vi "open-res-ra.vi"(7 "res-ra config":T1={"resource-type"="battery", "ra-ip"="127.0.0.1", "write-port"=32011, "listen-port"=32001}) -> (0 "error out":errorcluster, 5 "connection ID":refnum<k16>)   [LabVIEW 2021]
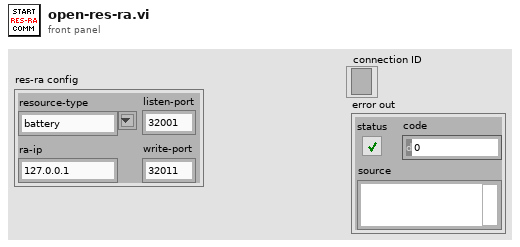
[diagram p1: front panel]
types:
  T1 = cluster{"resource-type":string, "ra-ip":string, "write-port":u16, "listen-port":u16}
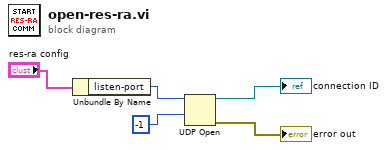
[diagram p0: block diagram]
diagram:
  n1 = Unbundle By Name("res-ra config") -> ("listen-port"=w3:u16)
  n2 = UDP Open(9:-1 ("timeout ms (25000)"), 11:w3) -> (port=→"connection ID":refnum<k16>, 0:→"error out":errorcluster)  [unwired: 3 in, 1 out]
